vi "PXI_Host_U64_Read_NewMethod_Benchmark.vi"() -> ()   [LabVIEW 2018]
uses:
  cRIO RT/FPGA Bitfile Register Operations/Scalar IO Operations/Read Methods/Read Data Register/Instances/Read U64.vi
  cRIO RT/FPGA Bitfile Register Operations/Scalar IO Operations/Utilities/Find Register Offset.vi
  cRIO RT/FPGA Bitfile Register Operations/Scalar IO Operations/SubVIs/Check Register Data Store.vi
  cRIO RT/FPGA Bitfile Register Operations/Scalar IO Operations/Error Handling/Error 6001.vi
  cRIO RT/FPGA Bitfile Register Operations/Scalar IO Operations/Error Handling/Error 6000.vi
  cRIO RT/FPGA Bitfile Register Operations/Scalar IO Operations/Error Handling/Error 6002.vi
  cRIO RT/FPGA Bitfile Register Operations/Scalar IO Operations/Error Handling/Error 6003.vi
  <vilib>/FPGAPlugInAG/Dynamic/niLvFpga_Close_Dynamic.vi
  <vilib>/rvi/interface/nirviCloseFPGA/nirviCloseFPGA.xnode
  cRIO RT/FPGA Bitfile Register Operations/Scalar IO Operations/FPGA Register IO.lvlib
panel:
  out "Value out":u64
  out "error out":errorcluster
  out "Execution time (s)":dbl
  # "Recorded time"
  # "3.37551E-5"
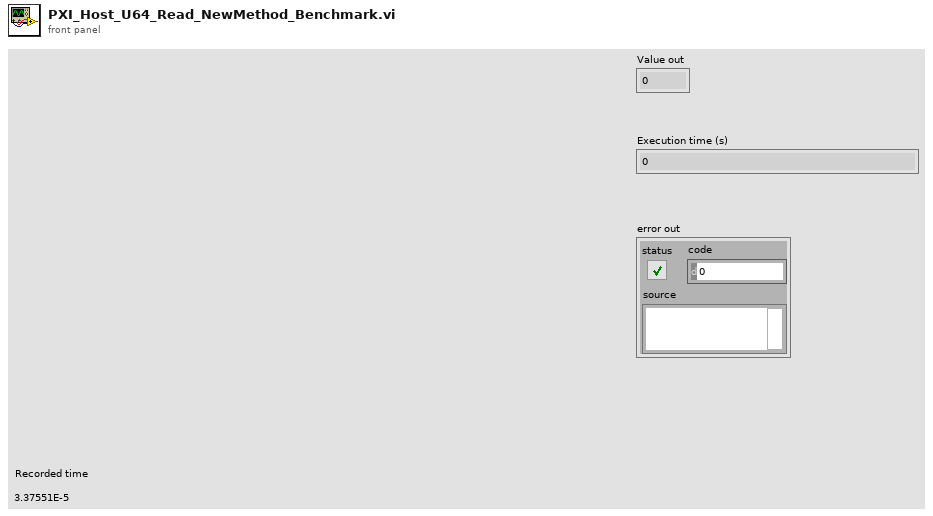
[diagram p1: front panel]
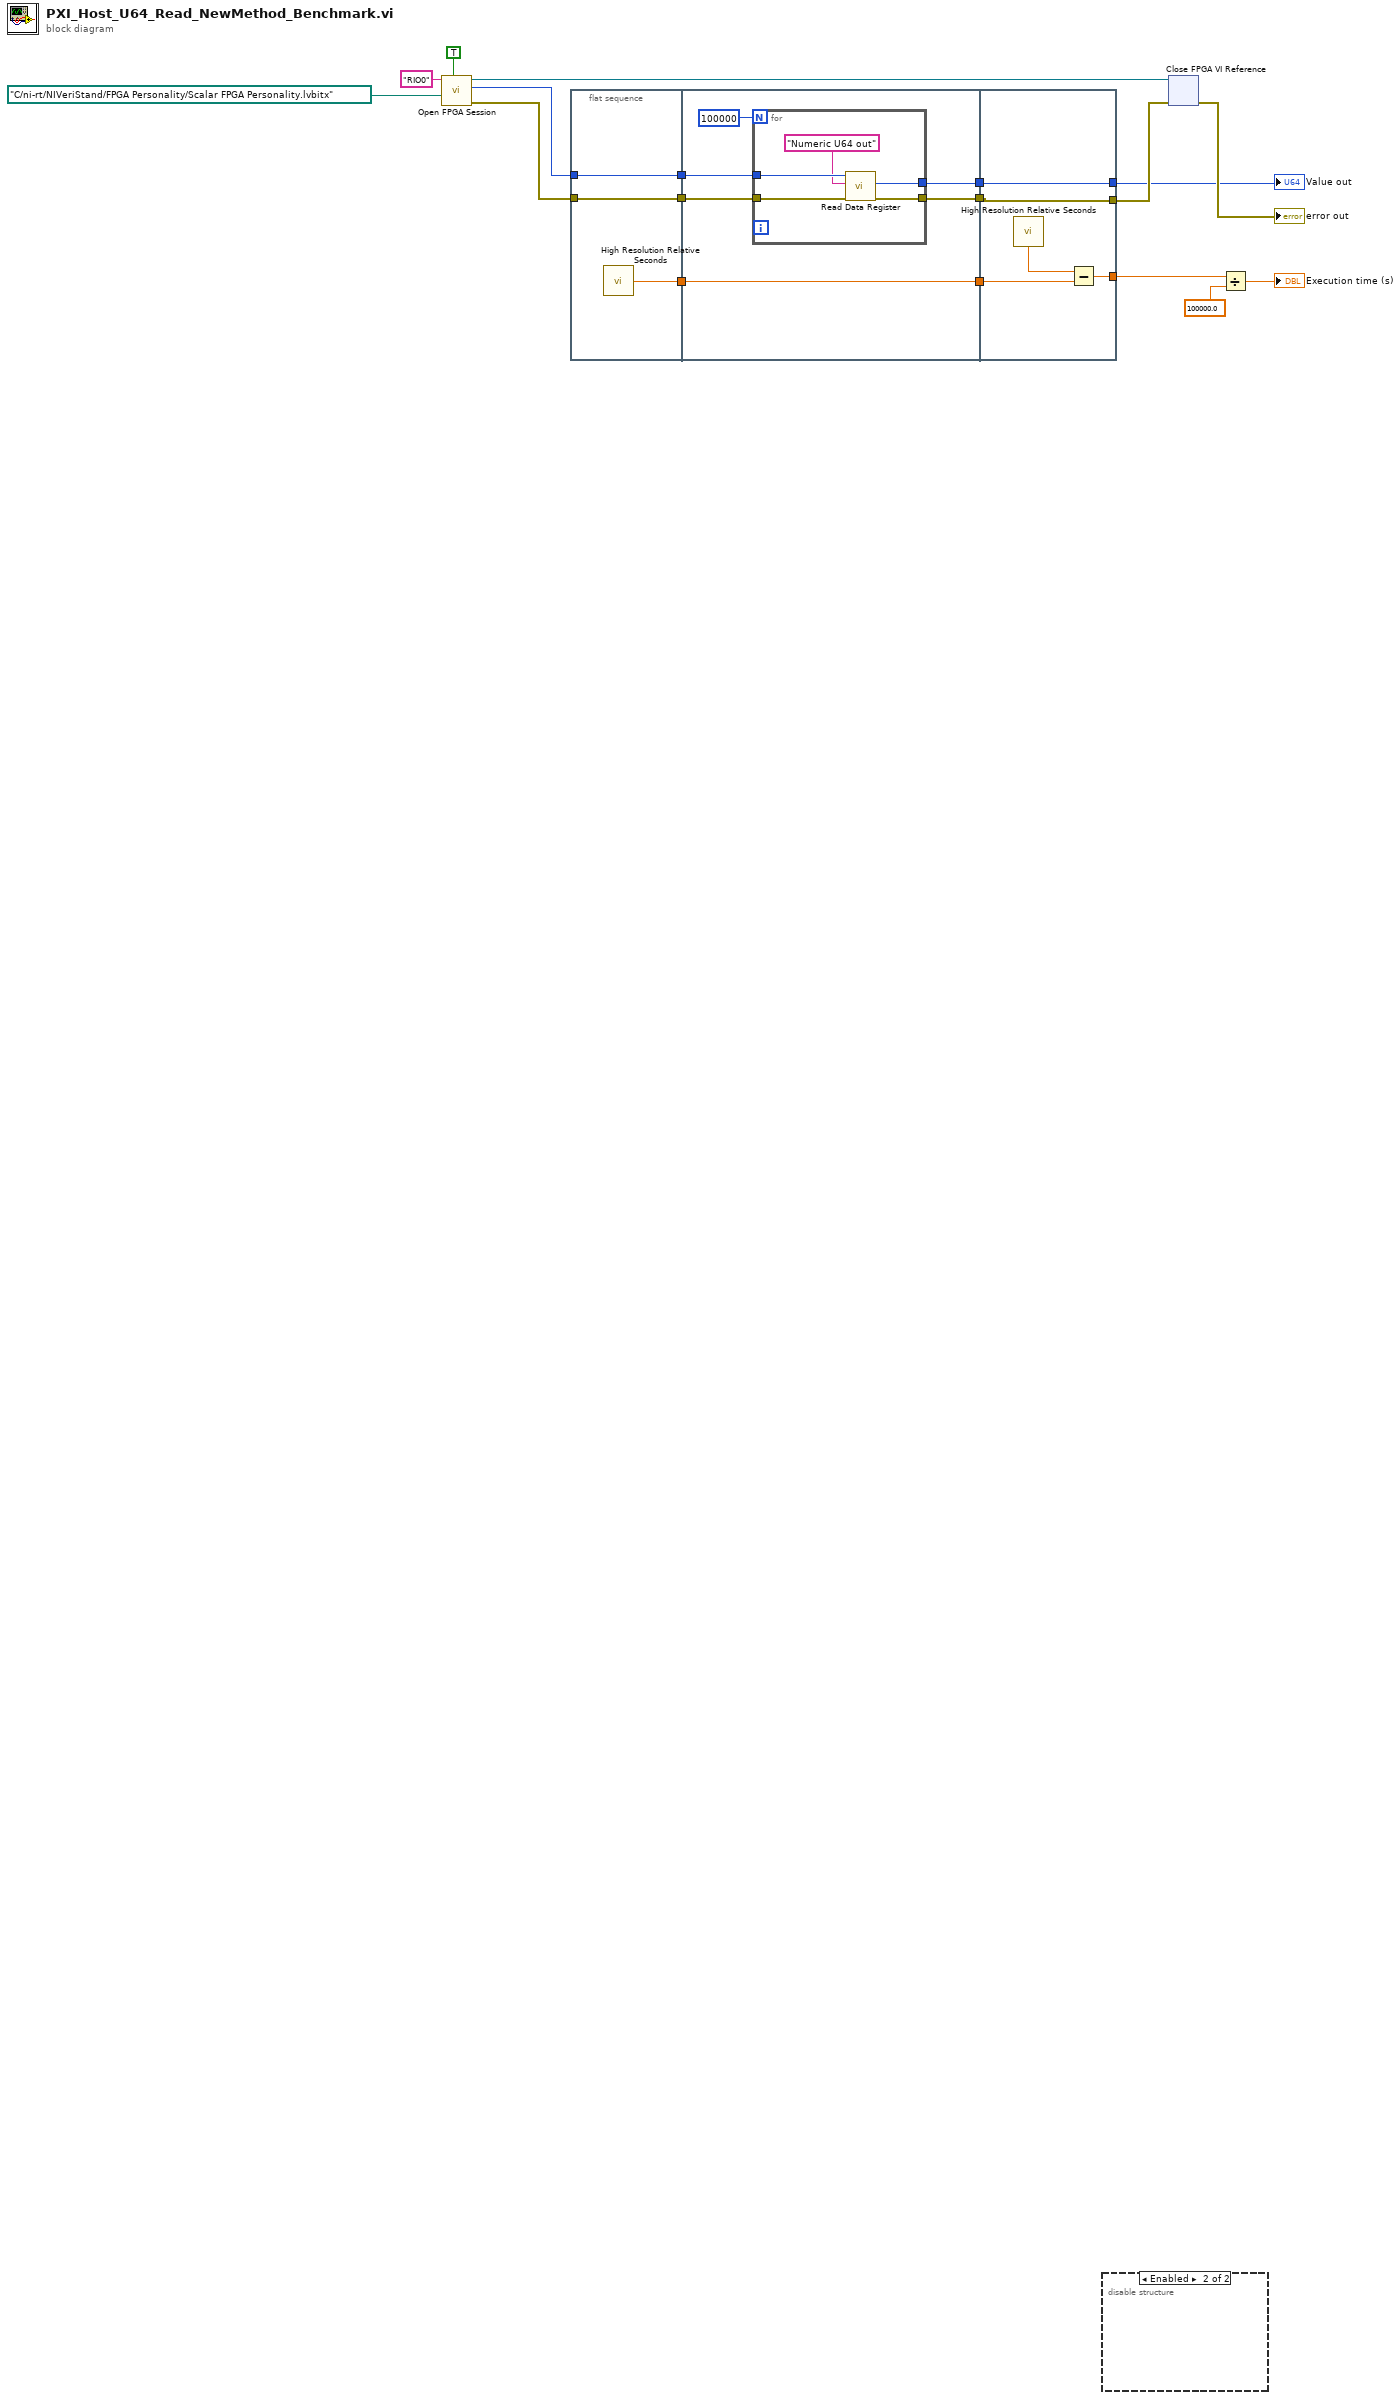
[diagram p0: block diagram]
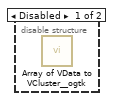
[diagram p2: hidden frame]
diagram:
  n1 = call "Open FPGA Session.vi"("run when loaded (T)"=TRUE, "bitfile path"=path "C:/ni-rt/NIVeriStand/FPGA Personality/Scalar FPGA Personality.lvbitx", "device address"="RIO0") -> ("error out"=w11:errorcluster, "session out"=w15:u32, "bitfile reference out"=w10:refnum<k20>)  [unwired: 6 in]
  n2 = flat-sequence {
    tunnel: [w21] -> w5
    tunnel: w15 -> [w20]
    tunnel: [w20] -> w4
    tunnel: w11 -> [w19]
    tunnel: [w19] -> w6
    tunnel: [w26] -> w3
    tunnel: w5 -> [w26]
    tunnel: w4 -> [w25]
    tunnel: w6 -> [w24]
    tunnel: [w23] -> w2
    tunnel: [w22] -> w1
    tunnel: w3 -> [w36]
    tunnel: [w35] -> w18
    tunnel: w2 -> [w34]
    tunnel: [w34] -> w9
    tunnel: w1 -> [w33]
    tunnel: [w33] -> w7
    frame #0 {
      n3 = call <vilib>:"High Resolution Relative Seconds.vi"() -> ("relative seconds"=w21:dbl)
    }
    frame #1 {
      n4 = for {
        N: 100000 -> [_]
        tunnel: w25 -> [w32]
        tunnel: w24 -> [w30]
        tunnel: [w28] -> w23
        tunnel: [w29] -> w22
        n5 = call-poly "Read Data Register.vi"("error in"=w30, "register name"="Numeric U64 out", "session in"=w32) -> ("error out"=w28:errorcluster, "value out"=w29:u64)  [unwired: 6 in, 1 out]
      }
    }
    frame #2 {
      n6 = call <vilib>:"High Resolution Relative Seconds.vi"() -> ("relative seconds"=w37:dbl)
      n7 = Subtract(x=w37, y=w36) -> (x-y=w35:dbl)
    }
  }
  n8 = disable-structure shown="Enabled" {
    frame Disabled {
      n9 = call <userlib>:"Array of VData to VCluster__ogtk.vi"() -> ()  [unwired: 10 in, 2 out]
    }
    frame Enabled {
    }
  }
  n10 = xnode "Close FPGA VI Reference"("FPGA VI Reference In"=w10, "error in"=w9) -> ("error out"=→"error out":errorcluster)
  n11 = Divide(x=w18, y=100000.0) -> (x/y=→"Execution time (s)":dbl)
  "Value out" <- w7
